vi "Test.vi"() -> ()   [LabVIEW 2012, in "Display Panel.lvlib" / "Abstract Display.lvclass"]
uses:
  Abstract Display.lvclass
  Universal Display/Universal Display.lvclass
  Data Logger Display/Data Logger Display.lvclass
  <vilib>/ActorFramework/Message Queue/Message Queue.lvclass/Message Queue.ctl
  <vilib>/ActorFramework/Message Enqueuer/Message Priority.ctl
  Abstract Display Messages/Write time digit Msg/Write time digit Msg.lvclass/Write time digit Msg.ctl
  <vilib>/ActorFramework/Message Enqueuer/Message Enqueuer.lvclass/Message Enqueuer.ctl
  Power Meter Display Messages/Write Card# Msg/Write Card# Msg.lvclass/Write Card# Msg.ctl
  <vilib>/ActorFramework/Message Enqueuer/Enqueue.vi
  <vilib>/ActorFramework/Message Priority Queue/Priority Enqueue.vi
  Abstract Display Messages/Write time digit Msg/Write time digit Msg.lvclass
  Power Meter Display Messages/Write Card# Msg/Write Card# Msg.lvclass
  <vilib>/ActorFramework/Stop Msg/Stop Msg.lvclass
  <vilib>/ActorFramework/Message Queue/Message Queue.lvclass
  <vilib>/ActorFramework/Actor/Actor.lvclass
  <vilib>/ActorFramework/Message Enqueuer/Message Enqueuer.lvclass
panel:
  in  "Boolean":bool
  in  "Card#":dbl
  out "error out":errorcluster
  in  "Stop Button":bool
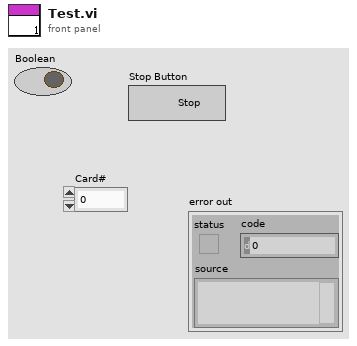
[diagram p1: front panel]
types:
  T1 = typedef "Actor Framework.lvlib/Message Enqueuer.lvclass/Message Priority.ctl" = enum16{"Low", "Normal", "High"}
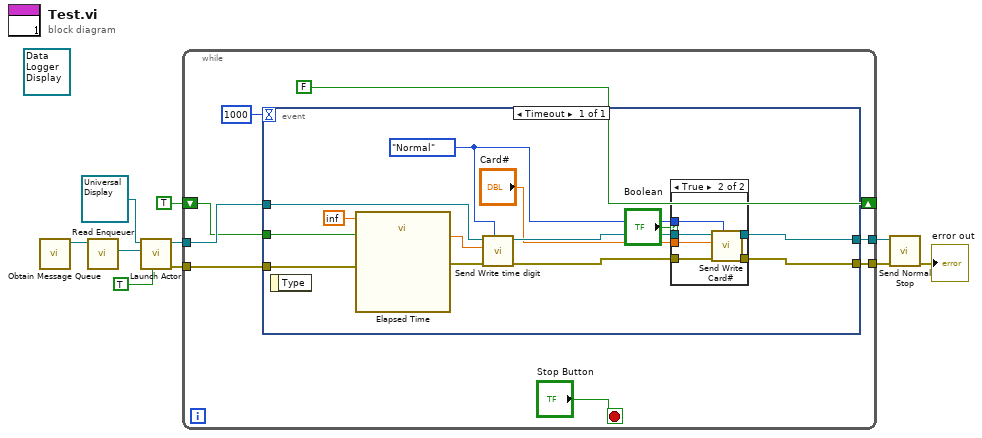
[diagram p0: block diagram]
diagram:
  (unwired) refnum<class "Data Logger Display.lvclass"> refnum ("Display Panel.lvlib:Data Logger Display.lvclass")
  n1 = call <vilib>:"Obtain Message Queue.vi"() -> ("Message Queue"=w10:refnum<class "Message Queue.lvclass">)  [unwired: 10 in, 1 out]
  n2 = call <vilib>:"Read Enqueuer.vi"("Message Queue"=w10) -> ("Message Enqueuer"=w9:refnum<class "Message Enqueuer.lvclass">)  [unwired: 10 in]
  n3 = call <vilib>:"Launch Actor.vi"("Open Actor Core front panel? (F)"=TRUE, "Actor-to-Caller Enqueuer"=w9, "Actor"=refnum<class "Universal Display.lvclass"> refnum ("Display Panel.lvlib:Universal Display.lvclass")) -> ("error out"=w6:errorcluster, "Caller-To-Actor Enqueuer"=w7:refnum<class "Message Enqueuer.lvclass">)  [unwired: 7 in]
  n4 = while {
    tunnel: w7 -> [w16]
    tunnel: [w15] -> w5
    tunnel: [w14] -> w4
    tunnel: w6 -> [w13]
    shift-right: [FALSE] -> _
    shift-left: TRUE -> [w12]
    stop <- "Stop Button" stop-if-true
    n5 = event shown="[0] Timeout" {
      selector: _ -> [_]
      dyn-events: _ -> [_]
      timeout: 1000 -> [_]
      tunnel: w16 -> [w26]
      tunnel: [w22] -> w15
      tunnel: [w23] -> w14
      tunnel: w13 -> [w27]
      tunnel: w12 -> [w30]
      event Timeout {
        w20 = Message_Priority."Normal" ("Message Priority (Normal)")
        n6 = event-data() -> ()  [unwired: 1 in, 1 out]
        n7 = call "Elapsed Time"("Time Target (s)"=inf, "Reset"=w30, "error in (no error)"=w27) -> ("Elapsed Time (s)"=w29:dbl, "error out"=w28:errorcluster)  [unwired: 9 in, 6 out]
        n8 = call "Send Write time digit.vi"("Message Priority (Normal)"=w20, "error in (no error)"=w28, "Time"=w29, "Message Enqueuer"=w26) -> ("error out"=w24:errorcluster, "Message Enqueuer out"=w25:refnum<class "Message Enqueuer.lvclass">)  [unwired: 6 in]
        n9 = case shown="True" "Boolean" {
          tunnel: w25 -> [w33 w39]
          tunnel: w24 -> [w32 w38]
          tunnel: [w32 w37] -> w23
          tunnel: [w33 w36] -> w22
          tunnel: "Card#" -> [_ w35]
          tunnel: w20 -> [_ w34]
          frame False {
          }
          frame True {
            n10 = call "Send Write Card#.vi"("Message Priority (Normal)"=w34, "error in (no error)"=w38, "Card#"=w35, "Message Enqueuer"=w39) -> ("error out"=w37:errorcluster, "Message Enqueuer out"=w36:refnum<class "Message Enqueuer.lvclass">)  [unwired: 6 in]
          }
        }
      }
    }
  }
  n11 = call <vilib>:"Send Normal Stop.vi"("error in (no error)"=w4, "Message Enqueuer"=w5) -> ("error out"=→"error out":errorcluster)  [unwired: 9 in]
